vi "Error Handling Test.vi"(10 "Error Code":dbl, 11 "Error Message":string) -> (3 "error out":errorcluster)   [LabVIEW 2024]
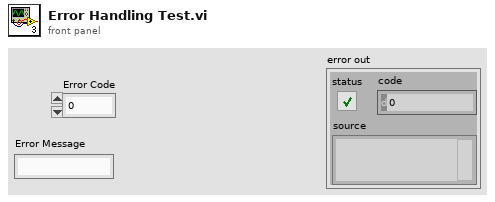
[diagram p1: front panel]
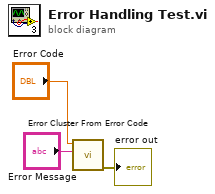
[diagram p0: block diagram]
diagram:
  n1 = call <vilib>:"Error Cluster From Error Code.vi"("error message (\"\")"="Error Message", "error code (0)"="Error Code") -> ("error out"=→"error out":errorcluster)  [unwired: 7 in]
